vi "target.vi"   [LabVIEW 2020]
uses:
  <vilib>/rvi/interface/RandomDataEmulation/niFpgaRandomDataHandleErrors.vi
  cholesky_decomposition_VIs/20_10_cholesky_decomposition.vi
  <vilib>/rvi/DataTransferAndStorage/Container/XNode/niFpgaContainer.xnode
  <vilib>/rvi/interface/RandomDataEmulation/nirviRandomDataFpgaReadWriteTemplate.vi
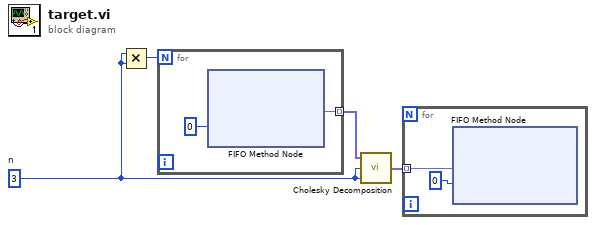
[diagram p0: block diagram]
diagram:
  w2 = 3  # n
  n1 = Multiply(x=w2, y=w2) -> (x*y=w1:i32)
  n2 = for {
    N: w1 -> [_]
    tunnel: [w6] -> w4 mode=indexing
    n3 = xnode ("FIFO Method Node")("Timeout"=0) -> ("Element"=w6:fxp<+/-,20,10>)  [unwired: 1 in, 2 out]
  }
  n4 = call-poly "Cholesky Decomposition.vi"("n"=w2, "m"=w2, "A"=w4) -> ("L"=w3:fxp<+/-,20,10>[])
  n5 = for {
    tunnel: w3 -> [w7] mode=indexing
    n6 = xnode ("FIFO Method Node")("Element"=w7, "Timeout"=0) -> ()  [unwired: 1 in, 2 out]
  }
